vi "AndorAdjustSliderRange.vi"(7 "AndorHistRange":refnum<vi>, 8 "error in (no error)":errorcluster, 9 "Imaq In":T1, 11 "Refnum in":T1) -> (0 "error out":errorcluster, 3 "Refnum out":T1)   [LabVIEW 2018, in "AndorOWN.lvlib"]
uses:
  AndorOWN.lvlib
  <vilib>/vision/Image Controls.llb/IMAQ Image.ctl
  <vilib>/vision/NI_Vision_Development_Module.lvlib
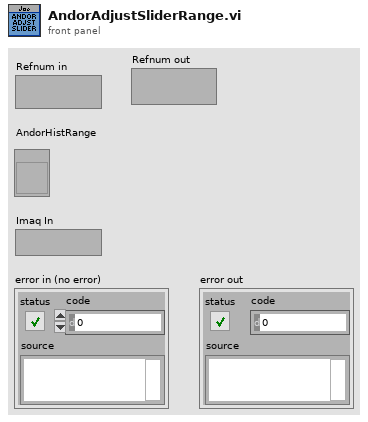
[diagram p1: front panel]
types:
  T1 = typedef "IMAQ Image.ctl" = refnum<image>
  T2 = enum32{"Linear", "Log", "Exp", "Square", "Square root", "Power X", "Power 1/X"}
  T3 = cluster{"histogram":u32[], "Minimal Value":sgl, "Maximal Value":sgl, "Starting Value":sgl, "Interval Width":sgl, "Mean Value":sgl, "Standard  Variation":sgl, "Area (pixels)":i32}
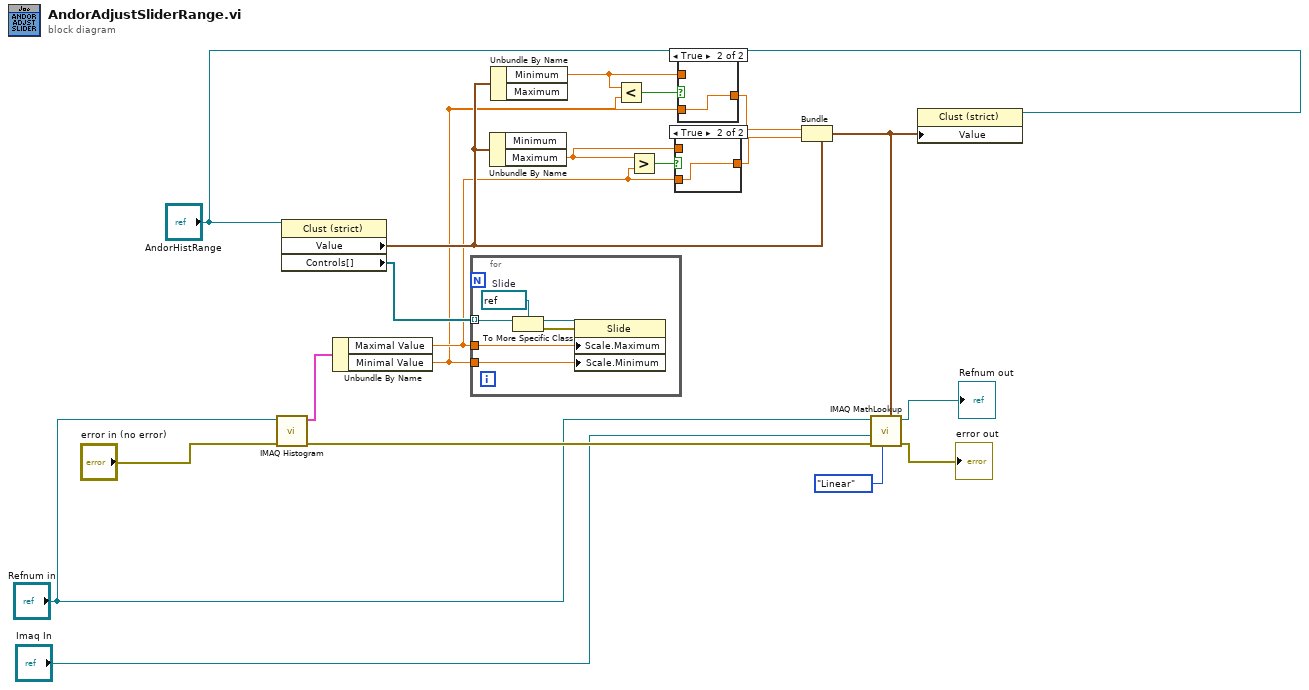
[diagram p0: block diagram]
diagram:
  n1 = call "IMAQ Histogram"("error in (no error)"="error in (no error)", "Image"="Refnum in") -> ("error out"=w12:errorcluster, "Histogram Report"=w9:T3)  [unwired: 8 in]
  n2 = property on="Property Node" class="Clust (strict)"(reference="AndorHistRange") -> ("Value"=w4:cluster{"Minimum":sgl, "Maximum":sgl}, "Controls[]"=w20:refnum<vi>[])  [unwired: 1 in, 2 out]
  n3 = Unbundle By Name(w9) -> ("Maximal Value"=w2:sgl, "Minimal Value"=w1:sgl)
  n4 = for {
    tunnel: w20 -> [w26] mode=indexing
    tunnel: w2 -> [w22]
    tunnel: w1 -> [w21]
    w25 = refnum<vi> refnum  # Slide
    n5 = To More Specific Class(target class=w25, reference=w26) -> (specific class reference=w24:refnum<vi>, error out=w23:errorcluster)  [unwired: 1 in]
    n6 = property class="Slide"(reference=w24, error in=w23, "Scale.Maximum"=w22, "Scale.Minimum"=w21) -> ()  [unwired: 2 out]
  }
  n7 = Unbundle By Name(w4) -> ("Maximum"=w3:sgl)  [unwired: 1 out]
  n8 = Unbundle By Name(w4) -> ("Minimum"=w14:sgl)  [unwired: 1 out]
  n9 = Less?(x=w14, y=w1) -> (x < y?=w13:bool)
  n10 = Greater?(x=w3, y=w2) -> (0:w17:bool)
  n11 = case shown="True" w17 {
    tunnel: w2 -> [_ w28]
    tunnel: [w27 w28] -> w16
    tunnel: w3 -> [w27 _]
    frame False {
    }
    frame True {
    }
  }
  n12 = case shown="True" w13 {
    tunnel: w1 -> [_ w30]
    tunnel: [w29 w30] -> w15
    tunnel: w14 -> [w29 _]
    frame False {
    }
    frame True {
    }
  }
  n13 = Bundle(cluster=w4, "Minimum"=w15, "Maximum"=w16) -> (w19:cluster{"Minimum":sgl, "Maximum":sgl})
  n14 = call "IMAQ MathLookup"("Range"=w19, "Operator"=T2."Linear", "error in (no error)"=w12, "Image Dst"="Imaq In", "Image Src"="Refnum in") -> ("error out"=→"error out":errorcluster, "Image Dst Out"=→"Refnum out":T1)  [unwired: 5 in]
  n15 = property class="Clust (strict)"(reference="AndorHistRange", "Value"=w19) -> ()  [unwired: 1 in, 2 out]
